vi "Pyramid_Reference.vi"(6 "Reference path":dbl[][](array[numeric]), 8 "interpolate":dbl, 9 "Refernce_logical":dbl[](array[numeric]), 10 "reference_corners":dbl[][](array[numeric]), 11 "corners_logical":dbl[](array[numeric])) -> ()   [LabVIEW 2015]
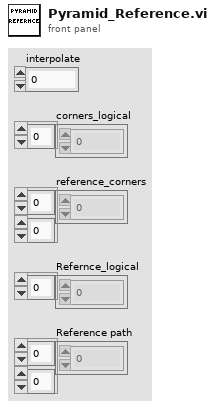
[diagram p1: front panel]
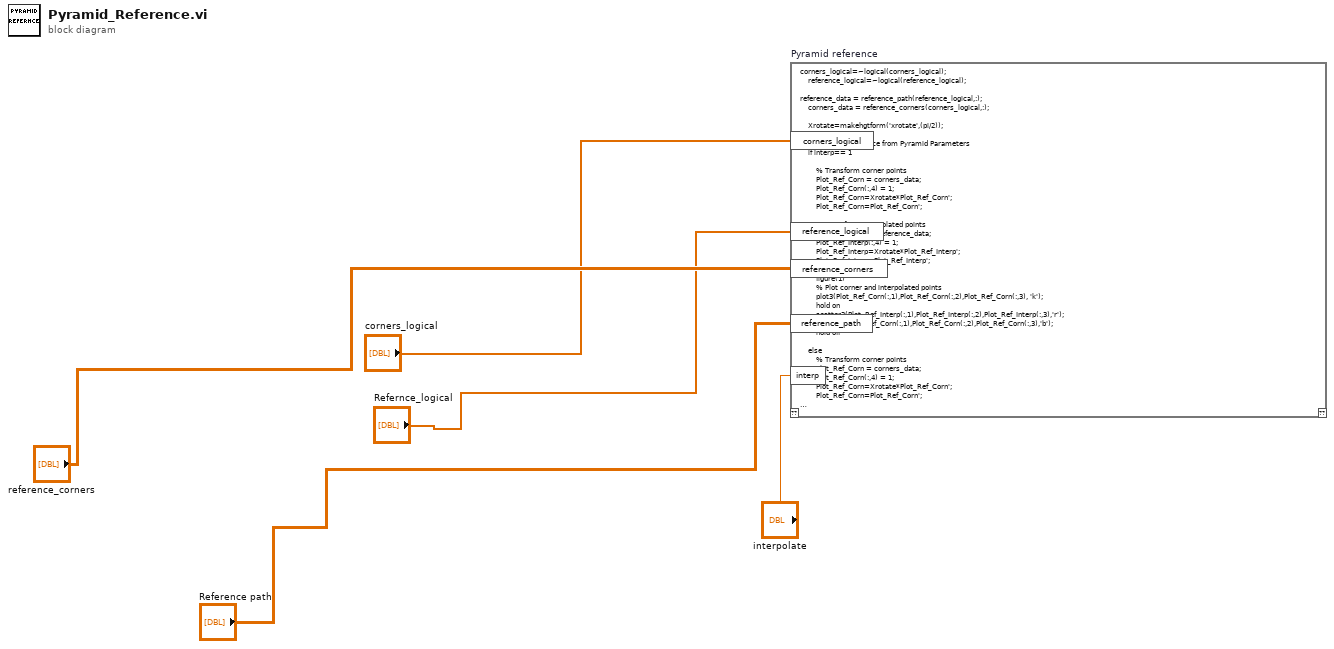
[diagram p0: block diagram]
diagram:
  n1 = script code="corners_logical=~logical(corners_logical);\n    reference_logical=~logical(reference_logical);\n\nreference_data = reference_path(reference_logical,:);\n    corners_data = reference_corners(corners_logical,:);\n    \n    Xrotate=makehgtform('xrotate',(pi/2));\n\n    %%% Plot Reference from Pyramid Parameters\n    if interp== 1\n                \n        % Transform corner points\n        Plot_Ref_Corn = corners_data;\n        Plot_Ref_Corn(:,4) = 1;\n        Plot_Ref_Corn=Xrotate*Plot_Ref_Corn';\n        Plot_Ref_Corn=Plot_Ref_Corn';\n        \n        % Transform interpolated points \n        Plot_Ref_Interp = reference_data;\n        Plot_Ref_Interp(:,4) = 1;\n        Plot_Ref_Interp=Xrotate*Plot_Ref_Interp';\n        Plot_Ref_Interp=Plot_Ref_Interp';\n        \n        figure(1)\n        % Plot corner and interpolated points\n        plot3(Plot_Ref_Corn(:,1),Plot_Ref_Corn(:,2),Plot_Ref_Corn(:,3), 'k');\n        hold on        \n        scatter3(Plot_Ref_Interp(:,1),Plot_Ref_Interp(:,2),Plot_Ref_Interp(:,3),'r');\n        scatter3(Plot_Ref_Corn(:,1),Plot_Ref_Corn(:,2),Plot_Ref_Corn(:,3),'b');\n        hold off\n        \n    else \n        % Transform corner points\n        Plot_Ref_Corn = corners_data;\n        Plot_Ref_Corn(:,4) = 1;\n        Plot_Ref_Corn=Xrotate*Plot_Ref_Corn';\n        Plot_Ref_Corn=Plot_Ref_Corn';\n        \n        % Plot corner points\n        figure(1)\n        plot3(Plot_Ref_Corn(:,1),Plot_Ref_Corn(:,2),Plot_Ref_Corn(:,3),'k');\n        hold on  \n        scatter3(Plot_Ref_Corn(:,1),Plot_Ref_Corn(:,2),Plot_Ref_Corn(:,3),'b');\n        hold off\n    end\n    \n    xlabel(\"X (mm)\");\n    ylabel(\"Y (mm)\");\n    zlabel(\"Z (mm)\");" "Pyramid reference"("corners_logical"="corners_logical", "reference_logical"="Refernce_logical", "reference_corners"="reference_corners", "reference_path"="Reference path", "interp"="interpolate") -> ()  [unwired: 1 in, 1 out]
